vi "Create log path.vi"(6 "extension (tdms)":string="tdms", 8 "error in (no error)":errorcluster, 9 "time stamp":timestamp, 10 "Prefix":string="data_", 11 "Path to directory":path) -> (0 "error out":errorcluster, 3 "Path":path)   [LabVIEW 2020]
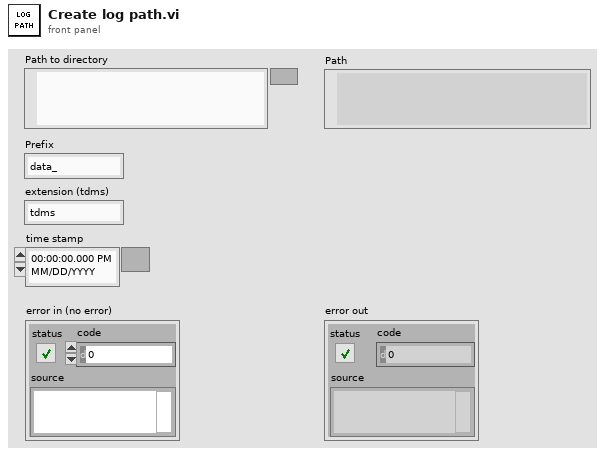
[diagram p1: front panel]
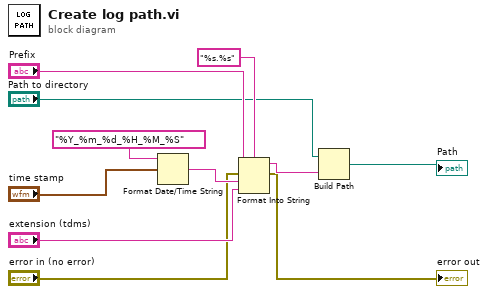
[diagram p0: block diagram]
diagram:
  n1 = Format Date/Time String(time format string (%c)="%Y_%m_%d_%H_%M_%S", seconds (now)="time stamp") -> (date/time string=w8:string)  [unwired: 1 in]
  n2 = Format Into String(format string="%s.%s", initial string="Prefix", error in="error in (no error)", w8, "extension (tdms)") -> (resulting string=w9:string, error out=→"error out":errorcluster)
  n3 = Build Path(base path="Path to directory", name or relative path=w9) -> (appended path=→"Path":path)
